vi "Fetch Single Record Single Channel(DBL).vi"(5 "FIFO Type":enum16{"FPGA to Host FIFO (U64)", "Generic"}(ring), 7 "Timeout (s)":i32=5, 8 "error in":errorcluster, 11 "FPGA VI Reference In":refnum<k20>) -> (0 "error out":errorcluster, 2 "Acquired Data":dbl[](array[numeric]) format="%.2f", 3 "FPGA VI Reference Out":refnum<k20>)   [LabVIEW 2011]
uses:
  <userlib>/FlexRIO Host Library/FlexRIO Host API/Acquire/Fetch/Fetch Acquired Data (U64).vi
  <vilib>/Utility/error.llb/Error Cluster From Error Code.vi
  <vilib>/rvi/errors/niLvFpgaAdjustHostInterfaceError.vi
  <vilib>/rvi/interface/nirviReadWriteControl/nirviReadWriteControl.xnode
  NiFpgaLv.dll
  <vilib>/rvi/interface/Simulation/niFpgaSimulationCallBeginRW.vi
  <userlib>/FlexRIO Host Library/FlexRIO Host Library (User).lvlib
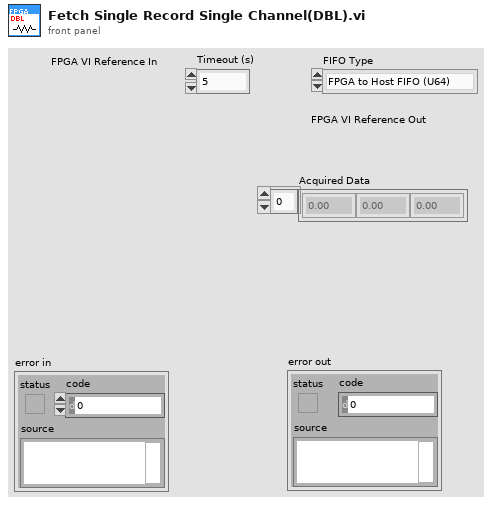
[diagram p1: front panel]
types:
  T1 = cluster{"Load Record Parameters?":bool, "Pre Trigger Samples":u16, "Samples per Record":u16, "Trigger Hold Off":u16, "Record Count":u16}
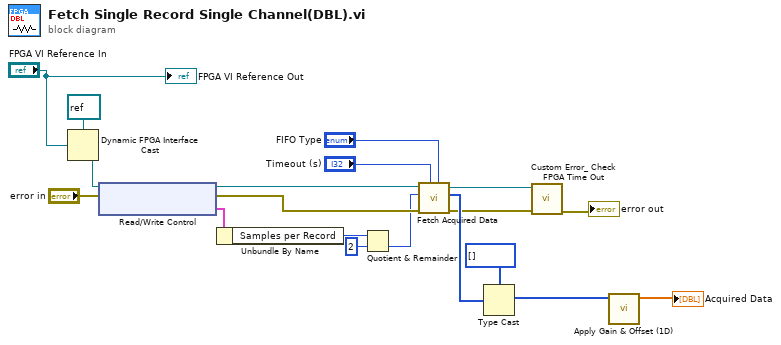
[diagram p0: block diagram]
diagram:
  n1 = Dynamic FPGA Interface Cast(Session In=refnum<k20> refnum ("Type"), Type="FPGA VI Reference In") -> (Session Out=w16:refnum<k20>)
  n2 = xnode "Read/Write Control"("FPGA VI Reference In"=w16, "error in"="error in") -> ("FPGA VI Reference Out"=w13:refnum<k20>, "error out"=w12:errorcluster, "Record Parameters"=w15:T1)
  n3 = Unbundle By Name(w15) -> ("Samples per Record"=w14:u16)
  n4 = Quotient & Remainder(x=w14, y=u16 2) -> (floor(x/y)=w1:u16)  [unwired: 1 out]
  n5 = call-poly <userlib>:"Fetch Acquired Data.vi"("FIFO Type"="FIFO Type", "Timeout (s)"="Timeout (s)", "error out"=w12, "Samples"=w1, "FPGA VI Reference In"=w13) -> ("error out"=w6:errorcluster, "Data"=w10:u64[], "FPGA VI Reference Out"=w7:refnum<k20>)  [unwired: 3 in, 1 out]
  n6 = Type Cast(type=i16[] [], x=w10) -> (*(type *) &x=w4:i16[])
  n7 = call <userlib>:"Custom Error_ Check FPGA Time Out.vi"("error in"=w6, "FPGA VI Reference In"=w7) -> ("error out"=→"error out":errorcluster)  [unwired: 8 in, 1 out]
  n8 = call <userlib>:"Apply Gain & Offset (1D).vi"("Raw Data"=w4) -> ("Scaled Data"=→"Acquired Data":dbl[])  [unwired: 10 in]
  "FPGA VI Reference Out" <- "FPGA VI Reference In"
